vi "GetRelativeCodePath.vi"(11 "Directory Name":string="CMCryoSysCode\\Matlab") -> (3 "appended path":path=path "C:/Code/CMCryoSysCode")   [LabVIEW 2017]
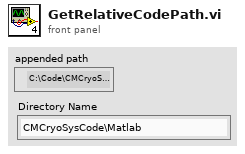
[diagram p1: front panel]
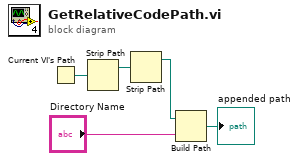
[diagram p0: block diagram]
diagram:
  n1 = Current VI's Path() -> (path=w2:path)
  n2 = Strip Path(path=w2) -> (stripped path=w3:path)  [unwired: 1 out]
  n3 = Strip Path(path=w3) -> (stripped path=w4:path)  [unwired: 1 out]
  n4 = Build Path(base path=w4, name or relative path="Directory Name") -> (appended path=→"appended path":path)
